vi "CAENHV Get Sys Prop Numeric.vi"(8 "error in (no error)":errorcluster, 10 "PropName":string, 11 "handle":i32) -> (0 "error out":errorcluster, 3 "Result":i16)   [LabVIEW 2018, in "CAENHVWrapper.lvlib"]
doc: "CAENHVLIB_API CAENHVRESULT CAENHV_GetSysProp(int handle, \n const char *PropName, void *Result);"
uses:
  <instrlib>/CAENHVWrapper/CAENHVWrapper.lvlib
  <instrlib>/CAENHVWrapper/VIs/CAENHVWrapper.dll
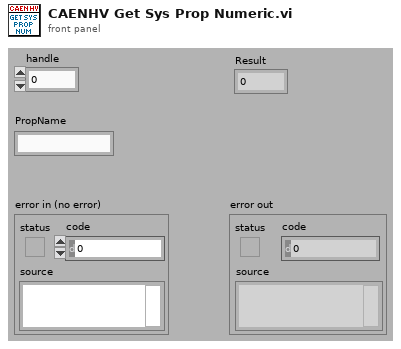
[diagram p1: front panel]
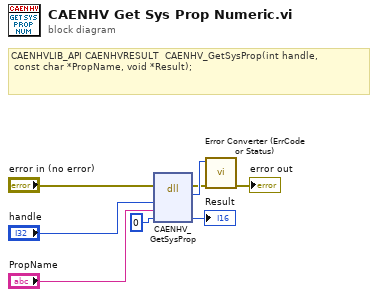
[diagram p0: block diagram]
diagram:
  # "CAENHVLIB_API CAENHVRESULT  CAENHV_GetSysProp(int handle, \n const char *PropName, void *Result);"
  n1 = dll-call lib="C:/Program Files (x86)/National Instruments/LabVIEW 2018/instr.lib/CAENHVWrapper/VIs/CAENHVWrapper.*" fn="CAENHV_GetSysProp"(error in="error in (no error)", "handle"="handle", "PropName"="PropName", "Result"=i16 0) -> (error out=w3:errorcluster, "return type"=w8:i32, "Result"=→"Result":i16)  [unwired: 4 in, 1 out]
  n2 = call <instrlib>:"Error Converter (ErrCode or Status).vi"("error in (no error)"=w3, "error code"=w8) -> ("error out"=→"error out":errorcluster)  [unwired: 9 in]
